vi "Save.vi"(8 "error in (no error)":errorcluster, 10 "Text":string, 11 "Experiment3D in":refnum<class "Experiment3D.lvclass">) -> (0 "error out":errorcluster, 3 "Experiment3D out":refnum<class "Experiment3D.lvclass">)   [LabVIEW 2014, in "Experiment3D.lvclass"]
uses:
  Experiment3D.lvclass
  Data/Data3D/Data3D.lvclass
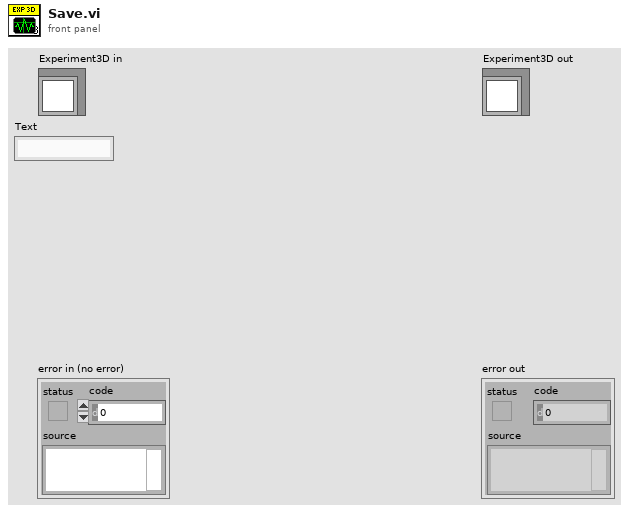
[diagram p1: front panel]
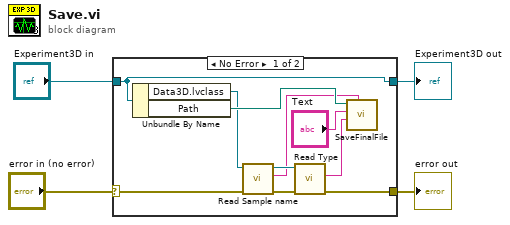
[diagram p0: block diagram]
diagram:
  n1 = case shown="No Error" "error in (no error)" {
    selector: "error in (no error)" -> [w7 w16]
    tunnel: [w5 w16] -> w3
    tunnel: [w14 w15] -> w1
    tunnel: "Experiment3D in" -> [w14 w15]
    frame No Error {
      n2 = Unbundle By Name(w14) -> ("Data3D.lvclass"=w12:refnum<class "Data3D.lvclass">, "Path"=w13:path)
      n3 = call "Read Sample name.vi"("error in (no error)"=w7, "Data3D in"=w12) -> ("error out"=w6:errorcluster, "Sample name"=w10:string, "Data3D out"=w11:refnum<class "Data3D.lvclass">)  [unwired: 7 in]
      n4 = call "Read Type.vi"("error in (no error)"=w6, "Data3D in"=w11) -> ("error out"=w5:errorcluster, "Type"=w9:string)  [unwired: 7 in, 1 out]
      n5 = call "SaveFinalFile.vi"("Sample name"=w10, "Type"=w9, "Text"="Text", "Path"=w13) -> ()  [unwired: 7 in, 1 out]
    }
    frame Error {
    }
  }
  "error out" <- w3
  "Experiment3D out" <- w1
